vi "from string.vi"(8 "error in":errorcluster, 9 "data":string, 10 "version":string, 11 "configuration in":refnum<class "Template Action Cfg.lvclass">) -> (0 "error out":errorcluster, 3 "configuration out":refnum<class "Template Action Cfg.lvclass">)   [LabVIEW 2014, in "Template Action Cfg.lvclass"]
doc: "Provides an interface for loading a module configuration from a file or other serialized data source. It is recommended that all children of this class store data in two sets--data required for its own initialization, and any data required for parent initialization--and that each implementation uses the <b>Call Parent Method</b> primitive to de-serialize parent information."
uses:
  Template Action Cfg.lvclass
  configuration data.ctl
  Template Action Cfg.lvclass/Template Action Cfg.ctl
  <vilib>/NI/TBM Modules/Sequencer/sequencer parent classes/action configuration parent/action configuration.lvclass
  <vilib>/NI/Configuration Framework/serializable configuration/NISE_CEF_serializable configuration.lvclass
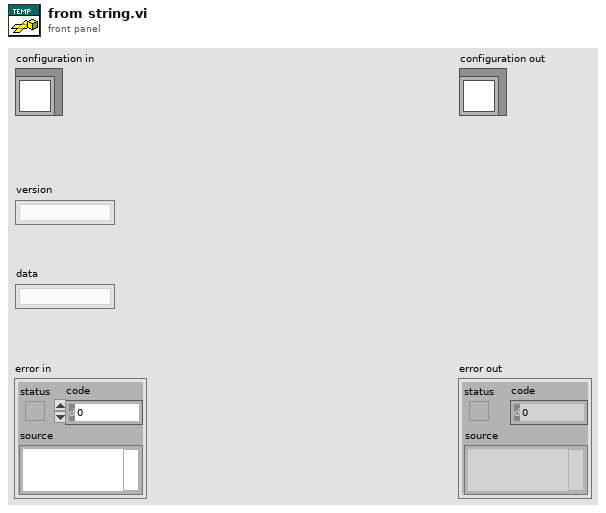
[diagram p1: front panel]
types:
  T1 = typedef "Template Action Cfg.lvclass/configuration data.ctl" = cluster{"Placeholder":dbl}
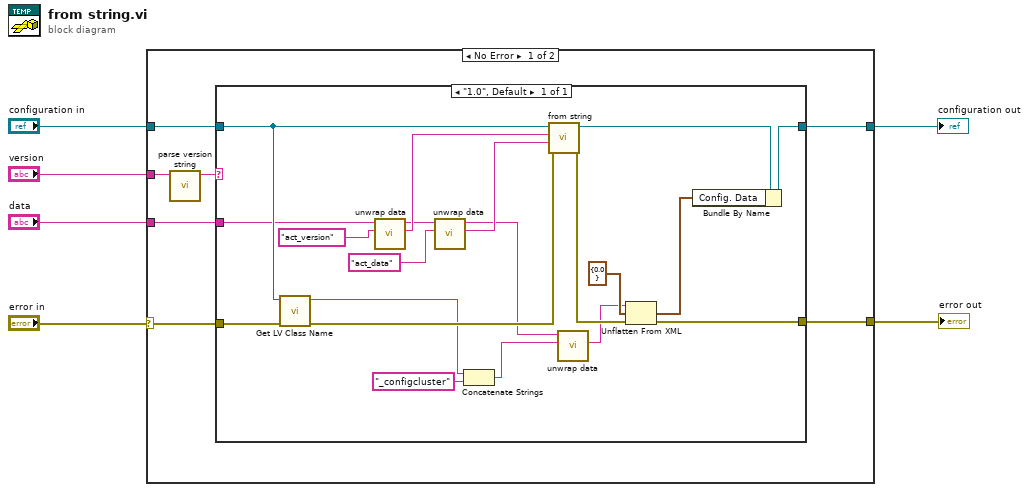
[diagram p0: block diagram]
diagram:
  n1 = case shown="No Error" "error in" {
    selector: "error in" -> [w10 w34]
    tunnel: "version" -> [w8 _]
    tunnel: "data" -> [w13 _]
    tunnel: "configuration in" -> [w12 w35]
    tunnel: [w11 w35] -> w2
    tunnel: [w9 w34] -> w1
    frame No Error {
      n2 = call <vilib>:"parse version string.vi"("full version"=w8) -> ("major.minor version"=w7:string)  [unwired: 7 in, 3 out]
      n3 = case shown="\"1.0\", Default" w7 {
        tunnel: w13 -> [w22]
        tunnel: w12 -> [w31]
        tunnel: [w32] -> w11
        tunnel: w10 -> [w30]
        tunnel: [w25] -> w9
        frame "1.0", Default {
          n4 = call <vilib>:"Get LV Class Name.vi"("error in (no error)"=w30, "object"=w31) -> ("error out"=w29:errorcluster, "class name"=w27:string)  [unwired: 8 in]
          n5 = call <vilib>:"unwrap data.vi"("identifier"="act_version" ("additional identifier"), "data to unwrap"=w22) -> ("unwrapped data"=w20:string, "remaining string"=w19:string)  [unwired: 8 in]
          n6 = call <vilib>:"unwrap data.vi"("identifier"="act_data" ("additional identifier"), "data to unwrap"=w19) -> ("unwrapped data"=w17:string, "remaining string"=w16:string)  [unwired: 8 in]
          n7 = Concatenate Strings(w27, "_configcluster" ("string")) -> (w15:string)
          n8 = call-parent "from string.vi"("error in"=w29, "data"=w17, "version"=w20, "configuration in"=w31) -> ("error out"=w26:errorcluster, "configuration out"=w33:refnum<class "Template Action Cfg.lvclass">)  [unwired: 6 in]
          n9 = call <vilib>:"unwrap data.vi"("identifier"=w15, "data to unwrap"=w16) -> ("unwrapped data"=w14:string)  [unwired: 8 in, 1 out]
          n10 = Unflatten From XML(xml string=w14, type=T1 {"Placeholder"=0.0} ("Config. Data"), error in (no error)=w26) -> (value=w23:T1, error out=w25:errorcluster)
          n11 = Bundle By Name(cluster=w33, "Config. Data"=w23) -> (w32:refnum<class "Template Action Cfg.lvclass">)
        }
      }
    }
    frame Error {
    }
  }
  "error out" <- w1
  "configuration out" <- w2
